vi "Fluke289.vi"(8 "error in (no error)":errorcluster, 11 "VISA resource name":refnum<visa-resource-name>) -> (0 "error out":errorcluster, 2 "Measurement":dbl format="%#_6f", 3 "VISA resource name out":refnum<visa-resource-name>)   [LabVIEW 2015, in "289.lvclass"]
uses:
  289.lvclass
panel:
  out "Unidad":string
  out "Read Buffer":string
  out "read buffer":string
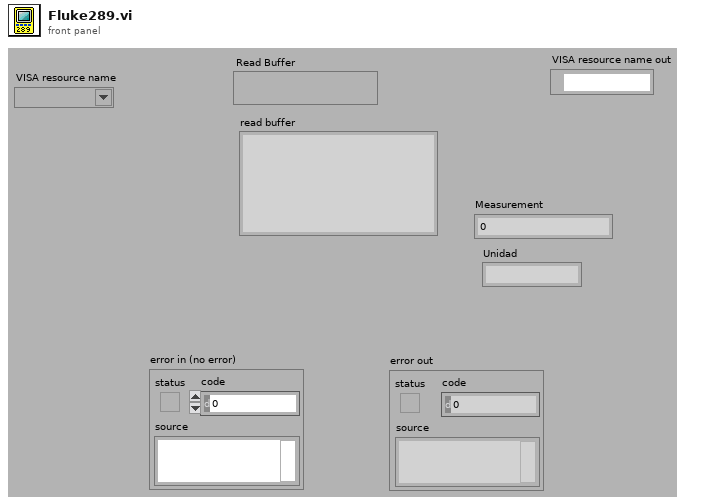
[diagram p1: front panel]
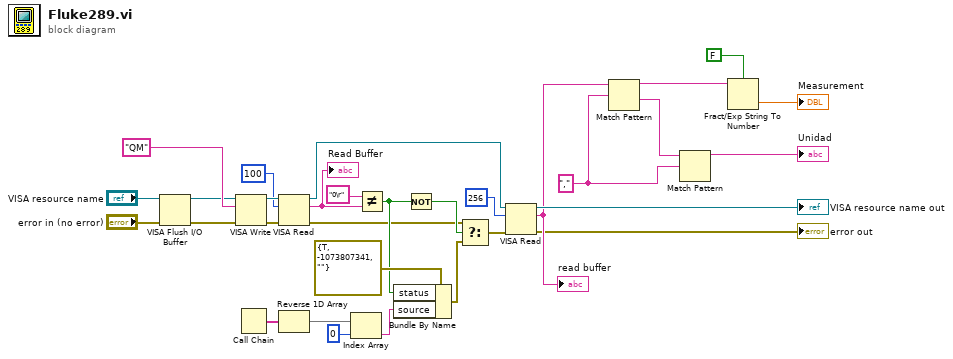
[diagram p0: block diagram]
diagram:
  w7 = "," ("regular expression")
  n1 = VISA Flush I/O Buffer(VISA resource name="VISA resource name", error in (no error)="error in (no error)") -> (VISA resource name out=w28:refnum<visa-resource-name>, error out=w27:errorcluster)  [unwired: 1 in]
  n2 = VISA Write(VISA resource name=w28, write buffer="QM" ("ID Query (QM)"), error in (no error)=w27) -> (VISA resource name out=w14:refnum<visa-resource-name>, error out=w12:errorcluster)  [unwired: 1 out]
  n3 = Call Chain() -> (call chain=w23:string[])
  n4 = VISA Read(VISA resource name=w14, byte count=u32 100 ("Byte Count (0)"), error in (no error)=w12) -> (VISA resource name out=w11:refnum<visa-resource-name>, read buffer=w19:string, error out=w15:errorcluster)  [unwired: 1 out]
  "Read Buffer" <- w19
  n5 = Reverse 1D Array(array=w23) -> (reversed array=w22:string[])
  n6 = Index Array(array=w22, index=0) -> (element=w21:string)
  n7 = Not Equal?(x="0\r", y=w19) -> (x != y?=w18:bool)
  n8 = Bundle By Name(cluster=errorcluster {"status"=TRUE, "code"=-1073807341, "source"=""} ("t"), "status"=w18, "source"=w21) -> (w16:errorcluster)
  n9 = Not(x=w18) -> (.not. x?=w17:bool)
  n10 = Select(t=w15, s=w17, f=w16) -> (s? t:f=w10:errorcluster)
  n11 = VISA Read(VISA resource name=w11, byte count=u32 256, error in (no error)=w10) -> (VISA resource name out=→"VISA resource name out":refnum<visa-resource-name>, read buffer=w9:string, error out=→"error out":errorcluster)  [unwired: 1 out]
  "read buffer" <- w9
  n12 = Match Pattern(string=w9, regular expression=w7) -> (before substring=w1:string, after substring=w8:string)  [unwired: 1 in, 2 out]
  n13 = Match Pattern(string=w8, regular expression=w7) -> (before substring=→"Unidad":string)  [unwired: 1 in, 3 out]
  n14 = Fract/Exp String To Number(use system decimal point (T)=FALSE, string=w1) -> (number=→"Measurement":dbl)  [unwired: 2 in, 1 out]
